vi "Data Check.vi"(0 "RFFE Command in":refnum<class "RFFE Command.lvclass">, 11 "error in (no error)":errorcluster) -> (4 "RFFE Command out":refnum<class "RFFE Command.lvclass">, 15 "error out":errorcluster)   [LabVIEW 2018, in "MIPI RFFE API.lvlib" / "RFFE Command.lvclass"]
uses:
  RFFE Command.lvclass
  RFFE Command.lvclass/RFFE Command.ctl
  Get Register Address.vi
  Get Slave Address.vi
  Get Register Address Limit.vi
  MIPI RFFE API.lvlib
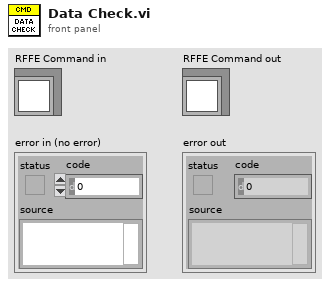
[diagram p1: front panel]
types:
  T1 = typedef "RFFE Commands.lvlib/Register Address.ctl" = u16
  T2 = typedef "RFFE Commands.lvlib/Slave Address.ctl" = u8
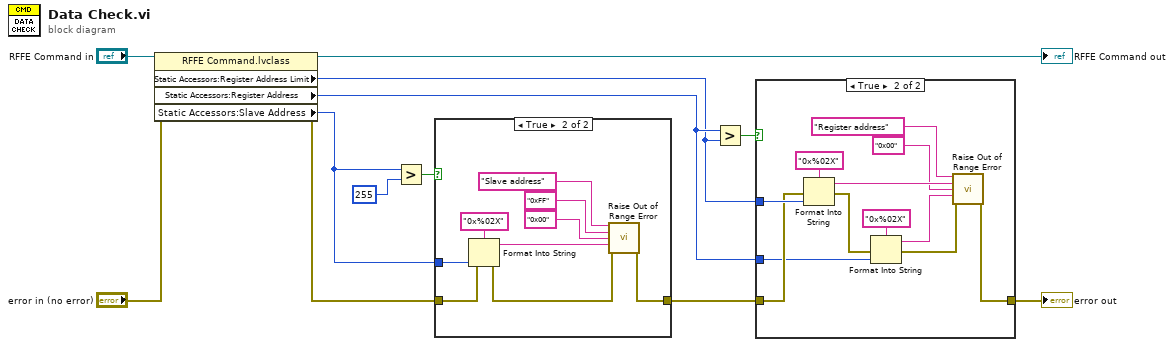
[diagram p0: block diagram]
diagram:
  n1 = property class="RFFE Command.lvclass"(reference="RFFE Command in", error in="error in (no error)") -> (reference out=→"RFFE Command out":refnum<class "RFFE Command.lvclass">, error out=w7:errorcluster, "Static Accessors:Register Address Limit"=w2:T1, "Static Accessors:Register Address"=w3:T1, "Static Accessors:Slave Address"=w6:T2)
  n2 = Greater?(x=w6, y=u8 255 ("upper limit")) -> (0:w4:bool)
  n3 = case shown="True" w4 {
    tunnel: w6 -> [_ w17]
    tunnel: w7 -> [w13 w15]
    tunnel: [w13 w20] -> w8
    frame False {
    }
    frame True {
      n4 = Format Into String(format string="0x%02X", error in=w15, w17) -> (resulting string=w14:string, error out=w16:errorcluster)  [unwired: 1 in]
      n5 = call "Raise Out of Range Error.vi"("Parameter Name"="Slave address", "Upper Limit"="0xFF" ("Lower Limit"), "Lower Limit"="0x00" ("Upper Limit"), "As Found"=w14, "error in (no error)"=w16) -> ("error out"=w20:errorcluster)  [unwired: 10 in]
    }
  }
  n6 = Greater?(x=w3, y=w2) -> (0:w1:bool)
  n7 = case shown="True" w1 {
    tunnel: w8 -> [w23 w28]
    tunnel: [w23 w35] -> w11
    tunnel: w3 -> [_ w27]
    tunnel: w2 -> [_ w32]
    frame False {
    }
    frame True {
      n8 = Format Into String(format string="0x%02X", error in=w28, w32) -> (resulting string=w25:string, error out=w30:errorcluster)  [unwired: 1 in]
      n9 = Format Into String(format string="0x%02X", error in=w30, w27) -> (resulting string=w26:string, error out=w29:errorcluster)  [unwired: 1 in]
      n10 = call "Raise Out of Range Error.vi"("Parameter Name"="Register address", "Upper Limit"=w25, "Lower Limit"="0x00", "As Found"=w26, "error in (no error)"=w29) -> ("error out"=w35:errorcluster)  [unwired: 10 in]
    }
  }
  "error out" <- w11
